vi "SubVI_Path2FigArray_001.vi"(1 "length (rest)":i32=3, 2 "paths":path[](array[path])) -> (0 "FIGS":string[](array[string]))   [LabVIEW 2018]
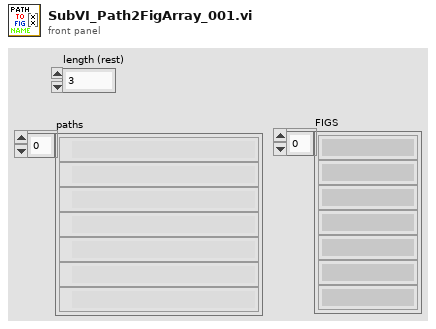
[diagram p1: front panel]
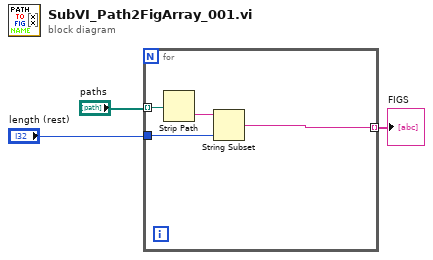
[diagram p0: block diagram]
diagram:
  n1 = for {
    tunnel: [w7] -> w3 mode=indexing
    tunnel: "paths" -> [w5] mode=indexing
    tunnel: "length (rest)" -> [w4]
    n2 = Strip Path(path=w5) -> (name=w6:string)  [unwired: 1 out]
    n3 = String Subset(string=w6, length (rest)=w4) -> (substring=w7:string)  [unwired: 1 in]
  }
  "FIGS" <- w3
